vi "MDrive_PollingReadParam.vi"(4 "Device Name":string, 6 "Mdrive Mode":T2, 8 "error in (no error)":errorcluster, 10 "Get Parameter":T1, 11 "VISA Refnum in":refnum<visa-resource-name>) -> (0 "error out":errorcluster, 1 "String":string, 2 "Value":i32, 3 "VISA Refnum out":refnum<visa-resource-name>)   [LabVIEW 2015]
uses:
  MDrive Mode.ctl
  Get Parameter.ctl
  Stream/LP Globals.vi
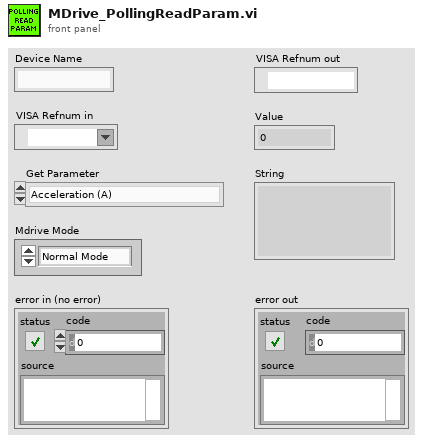
[diagram p1: front panel]
types:
  T1 = typedef "Get Parameter.ctl" = enum16{"Acceleration (A)", "Baud Rate (BD)", "Busy Flag (BY)", "Counter 1 (C1)", "Counter 2 (C2)", "Check Sum Enable (CK)", "Clock Mode (CM)", "Clock Mode Ratio (CR)", "Clock Mode Out Step Width (CW)", "Deceleration (D)", "Digital Filtering, Input 1 (D1)", "Digital Filtering, Input 2 (D2)", "Digital Filtering, Input 3 (D3)", "Digital Filtering, Input 4 (D4)", "Digital Filtering, Input 5 (D5)", "Digital Filtering, Input 9 (D9)", "Digital Filtering, Input 10 (D10)", "Digital Filtering, Input 11 (D11)", "Digital Filtering, Input 12 (D12)", "Deadband (DB)", "Enable/Disable Drive (DE)", "Device Name (DN)", "End Program Execution (E)", "Encoder Function Enable (EE)", "Encoder Lines (EL)", "Error Flag (EF)", "Error Variable (ER)", "Echo Mode (EM)", "Escape (ES)", "Execute Program at Address (EX)", "Hold Current (HC)", "Hold Current Delay Time (HI)", "Input 1 (I1)", "Input 2 (I2)", "Input 3 (I3)", "Input 4 (I4)", "Input 5 Analog (I5)", "Input 6 Encoder Index (I6)", "Input 9 (I9)", "Input 10 (I10)", "Input 11 (I11)", "Input 12 (I12)", "Input Low Byte (1-4) (IL)", "Input High Byte (9-12) (IH)", "Inputs Total (1-4,9-12) (IN)", "Internal Temperature (IT)", "Jog Enable (JE)", "Limit Stop Mode (LM)", "MicroStepping Select (MS)", "Motor Settling Delay Time (MT)", "Moving Flag (MV)", "Output 1 (O1)", "Output 2 (O2)", "Output 3 (O3)", "Output 4 (O4)", "Output 9 (O9)", "Output 10 (O10)", "Output 11 (O11)", "Output 12 (O12)", "Output High Byte (9-12) (OH)", "Output Low Byte (1-4) (OL)", "Output Total (1-4 and 9-12) (OT)", "Position (P)", "Position Captured at Trip (PC)", "Position Maintenance (PM)", "Part Number (PN)", "Party Mode (PY)", "Register 1 (R1)", "Register 2 (R2)", "Register 3 (R3)", "Register 4 (R4)", "Run Current (RC)", "Serial Number (SN)", "Stall Flag (ST)", "Stall Factor (SF)", "Stall Mode Set (SM)", "User Variables (UV)", "Velocity (V)", "Velocity Changing Flag (VC)", "Velocity Initial (VI)", "Version, Firmware (VR)", "Velocity Maximum (VM)", "Read Input1", "Read Input2"}
  T2 = typedef "MDrive Mode.ctl" = enum16{"Normal Mode", "Party Mode"}
  T3 = typedef "Semaphore RefNum" = refnum<k1>
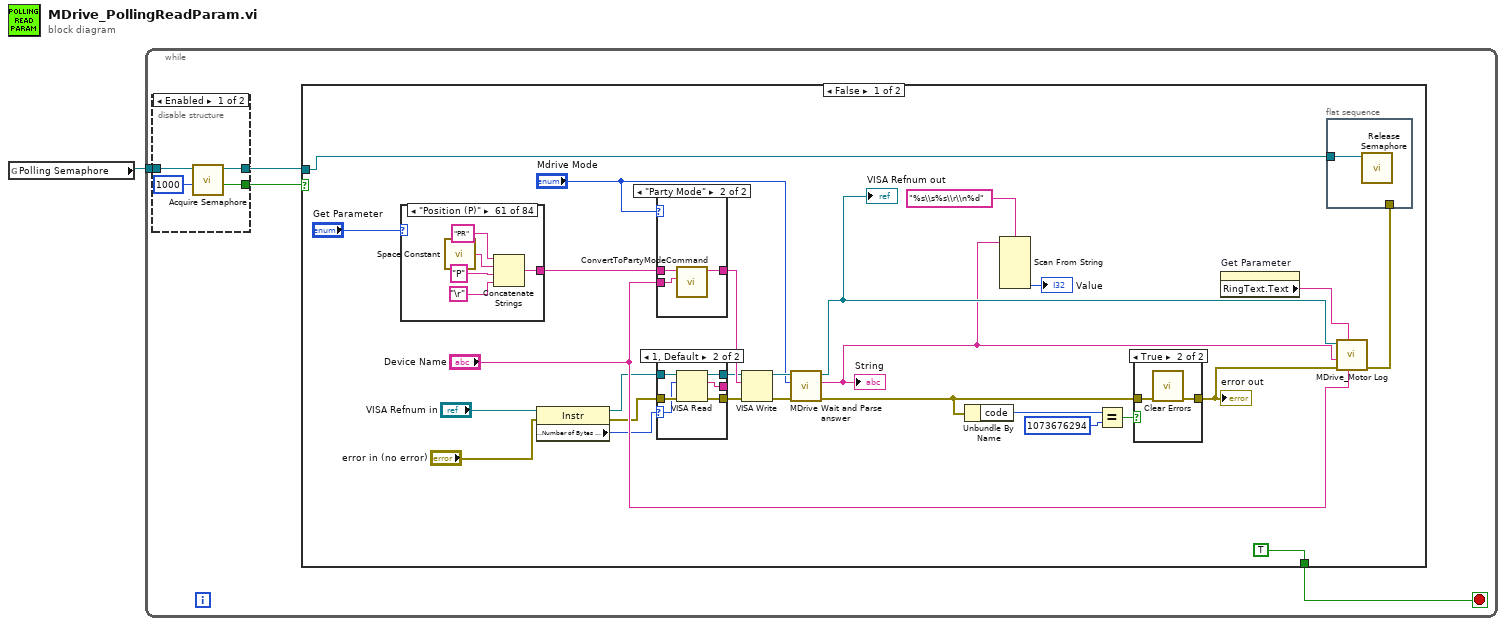
[diagram p0: block diagram]
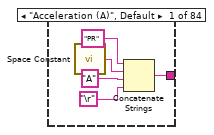
[diagram p5: hidden frame]
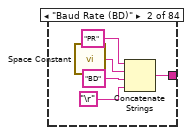
[diagram p6: hidden frame]
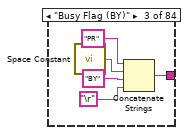
[diagram p7: hidden frame]
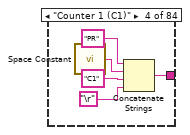
[diagram p8: hidden frame]
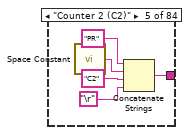
[diagram p9: hidden frame]
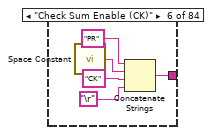
[diagram p10: hidden frame]
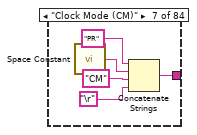
[diagram p11: hidden frame]
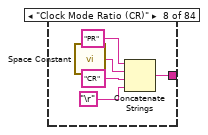
[diagram p12: hidden frame]
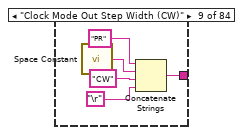
[diagram p13: hidden frame]
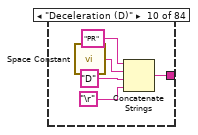
[diagram p14: hidden frame]
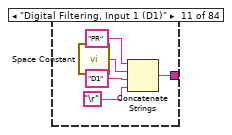
[diagram p15: hidden frame]
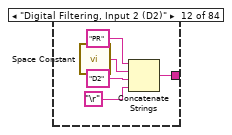
[diagram p16: hidden frame]
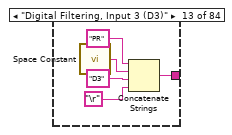
[diagram p17: hidden frame]
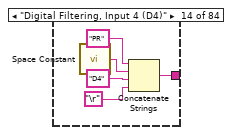
[diagram p18: hidden frame]
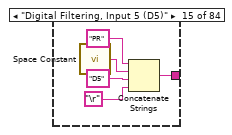
[diagram p19: hidden frame]
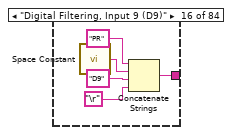
[diagram p20: hidden frame]
diagram:
  n1 = global read "LP Globals.vi" "Polling Semaphore"() -> (w1:T3)
  n2 = while {
    tunnel: w1 -> [w5]
    stop <- w4 stop-if-true
    n3 = disable-structure shown="Enabled" {
      disable-tunnel: w5 -> [w9 w10]
      disable-tunnel: [w7 w10] -> w3
      disable-tunnel: [w6 _] -> w2
      frame Enabled {
        n4 = call <vilib>:"Acquire Semaphore.vi"("ms timeout (-1)"=1000, "semaphore"=w9) -> ("timed out"=w6:bool, "semaphore out"=w7:T3)  [unwired: 3 in, 1 out]
      }
      frame Disabled {
      }
    }
    n5 = case shown="False" w2 {
      tunnel: [TRUE _] -> w4
      tunnel: w3 -> [w12 _]
      frame False {
        n6 = case shown="\"Position (P)\"" "Get Parameter" {
          tunnel: [w51 w56 w61 w66 w71 w76 w81 w86 w91 w96 w101 w106 w111 w116 w121 w126 w131 w136 w141 w146 w151 w156 w161 w166 w171 w176 w181 w186 w191 w196 w201 w206 w211 w216 w221 w226 w231 w236 w241 w246 w251 w256 w261 w266 w271 w276 w281 w286 w291 w296 w301 w306 w311 w316 w321 w326 w331 w336 w341 w346 w351 w356 w361 w366 w371 w376 w381 w386 w391 w396 w401 w406 w411 w416 w421 w426 w431 w436 w441 w446 w451 w456 w461 w466] -> w22
          frame "Acceleration (A)", Default {
            n7 = call <vilib>:"Space Constant.vi"() -> ("String"=w54:string)
            n8 = Concatenate Strings("PR" ("string"), w54, "A" ("string"), "\r") -> (w51:string)
          }
          frame "Baud Rate (BD)" {
            n9 = call <vilib>:"Space Constant.vi"() -> ("String"=w59:string)
            n10 = Concatenate Strings("PR" ("string"), w59, "BD" ("string"), "\r") -> (w56:string)
          }
          frame "Busy Flag (BY)" {
            n11 = call <vilib>:"Space Constant.vi"() -> ("String"=w64:string)
            n12 = Concatenate Strings("PR" ("string"), w64, "BY" ("string"), "\r") -> (w61:string)
          }
          frame "Counter 1 (C1)" {
            n13 = call <vilib>:"Space Constant.vi"() -> ("String"=w69:string)
            n14 = Concatenate Strings("PR" ("string"), w69, "C1" ("string"), "\r") -> (w66:string)
          }
          frame "Counter 2 (C2)" {
            n15 = call <vilib>:"Space Constant.vi"() -> ("String"=w74:string)
            n16 = Concatenate Strings("PR" ("string"), w74, "C2" ("string"), "\r") -> (w71:string)
          }
          frame "Check Sum Enable (CK)" {
            n17 = call <vilib>:"Space Constant.vi"() -> ("String"=w79:string)
            n18 = Concatenate Strings("PR" ("string"), w79, "CK" ("string"), "\r") -> (w76:string)
          }
          frame "Clock Mode (CM)" {
            n19 = call <vilib>:"Space Constant.vi"() -> ("String"=w84:string)
            n20 = Concatenate Strings("PR" ("string"), w84, "CM" ("string"), "\r") -> (w81:string)
          }
          frame "Clock Mode Ratio (CR)" {
            n21 = call <vilib>:"Space Constant.vi"() -> ("String"=w89:string)
            n22 = Concatenate Strings("PR" ("string"), w89, "CR" ("string"), "\r") -> (w86:string)
          }
          frame "Clock Mode Out Step Width (CW)" {
            n23 = call <vilib>:"Space Constant.vi"() -> ("String"=w94:string)
            n24 = Concatenate Strings("PR" ("string"), w94, "CW" ("string"), "\r") -> (w91:string)
          }
          frame "Deceleration (D)" {
            n25 = call <vilib>:"Space Constant.vi"() -> ("String"=w99:string)
            n26 = Concatenate Strings("PR" ("string"), w99, "D" ("string"), "\r") -> (w96:string)
          }
          frame "Digital Filtering, Input 1 (D1)" {
            n27 = call <vilib>:"Space Constant.vi"() -> ("String"=w104:string)
            n28 = Concatenate Strings("PR" ("string"), w104, "D1" ("string"), "\r") -> (w101:string)
          }
          frame "Digital Filtering, Input 2 (D2)" {
            n29 = call <vilib>:"Space Constant.vi"() -> ("String"=w109:string)
            n30 = Concatenate Strings("PR" ("string"), w109, "D2" ("string"), "\r") -> (w106:string)
          }
          frame "Digital Filtering, Input 3 (D3)" {
            n31 = call <vilib>:"Space Constant.vi"() -> ("String"=w114:string)
            n32 = Concatenate Strings("PR" ("string"), w114, "D3" ("string"), "\r") -> (w111:string)
          }
          frame "Digital Filtering, Input 4 (D4)" {
            n33 = call <vilib>:"Space Constant.vi"() -> ("String"=w119:string)
            n34 = Concatenate Strings("PR" ("string"), w119, "D4" ("string"), "\r") -> (w116:string)
          }
          frame "Digital Filtering, Input 5 (D5)" {
            n35 = call <vilib>:"Space Constant.vi"() -> ("String"=w124:string)
            n36 = Concatenate Strings("PR" ("string"), w124, "D5" ("string"), "\r") -> (w121:string)
          }
          frame "Digital Filtering, Input 9 (D9)" {
            n37 = call <vilib>:"Space Constant.vi"() -> ("String"=w129:string)
            n38 = Concatenate Strings("PR" ("string"), w129, "D9" ("string"), "\r") -> (w126:string)
          }
          frame "Digital Filtering, Input 10 (D10)" {
            n39 = call <vilib>:"Space Constant.vi"() -> ("String"=w134:string)
            n40 = Concatenate Strings("PR" ("string"), w134, "D10" ("string"), "\r") -> (w131:string)
          }
          frame "Digital Filtering, Input 11 (D11)" {
            n41 = call <vilib>:"Space Constant.vi"() -> ("String"=w139:string)
            n42 = Concatenate Strings("PR" ("string"), w139, "D11" ("string"), "\r") -> (w136:string)
          }
          frame "Digital Filtering, Input 12 (D12)" {
            n43 = call <vilib>:"Space Constant.vi"() -> ("String"=w144:string)
            n44 = Concatenate Strings("PR" ("string"), w144, "D12" ("string"), "\r") -> (w141:string)
          }
          frame "Deadband (DB)" {
            n45 = call <vilib>:"Space Constant.vi"() -> ("String"=w149:string)
            n46 = Concatenate Strings("PR" ("string"), w149, "DB" ("string"), "\r") -> (w146:string)
          }
          frame "Enable/Disable Drive (DE)" {
            n47 = call <vilib>:"Space Constant.vi"() -> ("String"=w154:string)
            n48 = Concatenate Strings("PR" ("string"), w154, "DE" ("string"), "\r") -> (w151:string)
          }
          frame "Device Name (DN)" {
            n49 = call <vilib>:"Space Constant.vi"() -> ("String"=w159:string)
            n50 = Concatenate Strings("PR" ("string"), w159, "DN" ("string"), "\r") -> (w156:string)
          }
          frame "End Program Execution (E)" {
            n51 = call <vilib>:"Space Constant.vi"() -> ("String"=w164:string)
            n52 = Concatenate Strings("PR" ("string"), w164, "E" ("string"), "\r") -> (w161:string)
          }
          frame "Encoder Function Enable (EE)" {
            n53 = call <vilib>:"Space Constant.vi"() -> ("String"=w169:string)
            n54 = Concatenate Strings("PR" ("string"), w169, "EE" ("string"), "\r") -> (w166:string)
          }
          frame "Error Flag (EF)" {
            n55 = call <vilib>:"Space Constant.vi"() -> ("String"=w174:string)
            n56 = Concatenate Strings("PR" ("string"), w174, "EF" ("string"), "\r") -> (w171:string)
          }
          frame "Error Variable (ER)" {
            n57 = call <vilib>:"Space Constant.vi"() -> ("String"=w179:string)
            n58 = Concatenate Strings("PR" ("string"), w179, "ER" ("string"), "\r") -> (w176:string)
          }
          frame "Echo Mode (EM)" {
            n59 = call <vilib>:"Space Constant.vi"() -> ("String"=w184:string)
            n60 = Concatenate Strings("PR" ("string"), w184, "EM" ("string"), "\r") -> (w181:string)
          }
          frame "Escape (ES)" {
            n61 = call <vilib>:"Space Constant.vi"() -> ("String"=w189:string)
            n62 = Concatenate Strings("PR" ("string"), w189, "ES" ("string"), "\r") -> (w186:string)
          }
          frame "Execute Program at Address (EX)" {
            n63 = call <vilib>:"Space Constant.vi"() -> ("String"=w194:string)
            n64 = Concatenate Strings("PR" ("string"), w194, "EX" ("string"), "\r") -> (w191:string)
          }
          frame "Hold Current (HC)" {
            n65 = call <vilib>:"Space Constant.vi"() -> ("String"=w199:string)
            n66 = Concatenate Strings("PR" ("string"), w199, "HC" ("string"), "\r") -> (w196:string)
          }
          frame "Hold Current Delay Time (HI)" {
            n67 = call <vilib>:"Space Constant.vi"() -> ("String"=w204:string)
            n68 = Concatenate Strings("PR" ("string"), w204, "HI" ("string"), "\r") -> (w201:string)
          }
          frame "Input 1 (I1)" {
            n69 = call <vilib>:"Space Constant.vi"() -> ("String"=w209:string)
            n70 = Concatenate Strings("PR" ("string"), w209, "I1" ("string"), "\r") -> (w206:string)
          }
          frame "Input 2 (I2)" {
            n71 = call <vilib>:"Space Constant.vi"() -> ("String"=w214:string)
            n72 = Concatenate Strings("PR" ("string"), w214, "I2" ("string"), "\r") -> (w211:string)
          }
          frame "Input 3 (I3)" {
            n73 = call <vilib>:"Space Constant.vi"() -> ("String"=w219:string)
            n74 = Concatenate Strings("PR" ("string"), w219, "I3" ("string"), "\r") -> (w216:string)
          }
          frame "Input 4 (I4)" {
            n75 = call <vilib>:"Space Constant.vi"() -> ("String"=w224:string)
            n76 = Concatenate Strings("PR" ("string"), w224, "I4" ("string"), "\r") -> (w221:string)
          }
          frame "Input 5 Analog (I5)" {
            n77 = call <vilib>:"Space Constant.vi"() -> ("String"=w229:string)
            n78 = Concatenate Strings("PR" ("string"), w229, "I5" ("string"), "\r") -> (w226:string)
          }
          frame "Input 6 Encoder Index (I6)" {
            n79 = call <vilib>:"Space Constant.vi"() -> ("String"=w234:string)
            n80 = Concatenate Strings("PR" ("string"), w234, "I6" ("string"), "\r") -> (w231:string)
          }
          frame "Input 9 (I9)" {
            n81 = call <vilib>:"Space Constant.vi"() -> ("String"=w239:string)
            n82 = Concatenate Strings("PR" ("string"), w239, "I9" ("string"), "\r") -> (w236:string)
          }
          frame "Input 10 (I10)" {
            n83 = call <vilib>:"Space Constant.vi"() -> ("String"=w244:string)
            n84 = Concatenate Strings("PR" ("string"), w244, "I10" ("string"), "\r") -> (w241:string)
          }
          frame "Input 11 (I11)" {
            n85 = call <vilib>:"Space Constant.vi"() -> ("String"=w249:string)
            n86 = Concatenate Strings("PR" ("string"), w249, "I3" ("string"), "\r") -> (w246:string)
          }
          frame "Input 12 (I12)" {
            n87 = call <vilib>:"Space Constant.vi"() -> ("String"=w254:string)
            n88 = Concatenate Strings("PR" ("string"), w254, "I12" ("string"), "\r") -> (w251:string)
          }
          frame "Input Low Byte (1-4) (IL)" {
            n89 = call <vilib>:"Space Constant.vi"() -> ("String"=w259:string)
            n90 = Concatenate Strings("PR" ("string"), w259, "IL" ("string"), "\r") -> (w256:string)
          }
          frame "Input High Byte (9-12) (IH)" {
            n91 = call <vilib>:"Space Constant.vi"() -> ("String"=w264:string)
            n92 = Concatenate Strings("PR" ("string"), w264, "IH" ("string"), "\r") -> (w261:string)
          }
          frame "Inputs Total (1-4,9-12) (IN)" {
            n93 = call <vilib>:"Space Constant.vi"() -> ("String"=w269:string)
            n94 = Concatenate Strings("PR" ("string"), w269, "IN" ("string"), "\r") -> (w266:string)
          }
          frame "Internal Temperature (IT)" {
            n95 = call <vilib>:"Space Constant.vi"() -> ("String"=w274:string)
            n96 = Concatenate Strings("PR" ("string"), w274, "IT" ("string"), "\r") -> (w271:string)
          }
          frame "Jog Enable (JE)" {
            n97 = call <vilib>:"Space Constant.vi"() -> ("String"=w279:string)
            n98 = Concatenate Strings("PR" ("string"), w279, "JE" ("string"), "\r") -> (w276:string)
          }
          frame "Limit Stop Mode (LM)" {
            n99 = call <vilib>:"Space Constant.vi"() -> ("String"=w284:string)
            n100 = Concatenate Strings("PR" ("string"), w284, "LM" ("string"), "\r") -> (w281:string)
          }
          frame "MicroStepping Select (MS)" {
            n101 = call <vilib>:"Space Constant.vi"() -> ("String"=w289:string)
            n102 = Concatenate Strings("PR" ("string"), w289, "MS" ("string"), "\r") -> (w286:string)
          }
          frame "Motor Settling Delay Time (MT)" {
            n103 = call <vilib>:"Space Constant.vi"() -> ("String"=w294:string)
            n104 = Concatenate Strings("PR" ("string"), w294, "MT" ("string"), "\r") -> (w291:string)
          }
          frame "Output 1 (O1)" {
            n105 = call <vilib>:"Space Constant.vi"() -> ("String"=w299:string)
            n106 = Concatenate Strings("PR" ("string"), w299, "O1" ("string"), "\r") -> (w296:string)
          }
          frame "Output 2 (O2)" {
            n107 = call <vilib>:"Space Constant.vi"() -> ("String"=w304:string)
            n108 = Concatenate Strings("PR" ("string"), w304, "O2" ("string"), "\r") -> (w301:string)
          }
          frame "Output 3 (O3)" {
            n109 = call <vilib>:"Space Constant.vi"() -> ("String"=w309:string)
            n110 = Concatenate Strings("PR" ("string"), w309, "O3" ("string"), "\r") -> (w306:string)
          }
          frame "Output 4 (O4)" {
            n111 = call <vilib>:"Space Constant.vi"() -> ("String"=w314:string)
            n112 = Concatenate Strings("PR" ("string"), w314, "O4" ("string"), "\r") -> (w311:string)
          }
          frame "Output 9 (O9)" {
            n113 = call <vilib>:"Space Constant.vi"() -> ("String"=w319:string)
            n114 = Concatenate Strings("PR" ("string"), w319, "O9" ("string"), "\r") -> (w316:string)
          }
          frame "Output 10 (O10)" {
            n115 = call <vilib>:"Space Constant.vi"() -> ("String"=w324:string)
            n116 = Concatenate Strings("PR" ("string"), w324, "O10" ("string"), "\r") -> (w321:string)
          }
          frame "Output 11 (O11)" {
            n117 = call <vilib>:"Space Constant.vi"() -> ("String"=w329:string)
            n118 = Concatenate Strings("PR" ("string"), w329, "O11" ("string"), "\r") -> (w326:string)
          }
          frame "Output 12 (O12)" {
            n119 = call <vilib>:"Space Constant.vi"() -> ("String"=w334:string)
            n120 = Concatenate Strings("PR" ("string"), w334, "O12" ("string"), "\r") -> (w331:string)
          }
          frame "Output High Byte (9-12) (OH)" {
            n121 = call <vilib>:"Space Constant.vi"() -> ("String"=w339:string)
            n122 = Concatenate Strings("PR" ("string"), w339, "OH" ("string"), "\r") -> (w336:string)
          }
          frame "Output Low Byte (1-4) (OL)" {
            n123 = call <vilib>:"Space Constant.vi"() -> ("String"=w344:string)
            n124 = Concatenate Strings("PR" ("string"), w344, "OL" ("string"), "\r") -> (w341:string)
          }
          frame "Output Total (1-4 and 9-12) (OT)" {
            n125 = call <vilib>:"Space Constant.vi"() -> ("String"=w349:string)
            n126 = Concatenate Strings("PR" ("string"), w349, "OT" ("string"), "\r") -> (w346:string)
          }
          frame "Position (P)" {
            n127 = call <vilib>:"Space Constant.vi"() -> ("String"=w354:string)
            n128 = Concatenate Strings("PR" ("string"), w354, "P" ("string"), "\r") -> (w351:string)
          }
          frame "Position Captured at Trip (PC)" {
            n129 = call <vilib>:"Space Constant.vi"() -> ("String"=w359:string)
            n130 = Concatenate Strings("PR" ("string"), w359, "PC" ("string"), "\r") -> (w356:string)
          }
          frame "Position Maintenance (PM)" {
            n131 = call <vilib>:"Space Constant.vi"() -> ("String"=w364:string)
            n132 = Concatenate Strings("PR" ("string"), w364, "PM" ("string"), "\r") -> (w361:string)
          }
          frame "Part Number (PN)" {
            n133 = call <vilib>:"Space Constant.vi"() -> ("String"=w369:string)
            n134 = Concatenate Strings("PR" ("string"), w369, "PN" ("string"), "\r") -> (w366:string)
          }
          frame "Party Mode (PY)" {
            n135 = call <vilib>:"Space Constant.vi"() -> ("String"=w374:string)
            n136 = Concatenate Strings("PR" ("string"), w374, "PY" ("string"), "\r") -> (w371:string)
          }
          frame "Register 1 (R1)" {
            n137 = call <vilib>:"Space Constant.vi"() -> ("String"=w379:string)
            n138 = Concatenate Strings("PR" ("string"), w379, "R1" ("string"), "\r") -> (w376:string)
          }
          frame "Register 2 (R2)" {
            n139 = call <vilib>:"Space Constant.vi"() -> ("String"=w384:string)
            n140 = Concatenate Strings("PR" ("string"), w384, "R2" ("string"), "\r") -> (w381:string)
          }
          frame "Register 3 (R3)" {
            n141 = call <vilib>:"Space Constant.vi"() -> ("String"=w389:string)
            n142 = Concatenate Strings("PR" ("string"), w389, "R3" ("string"), "\r") -> (w386:string)
          }
          frame "Register 4 (R4)" {
            n143 = call <vilib>:"Space Constant.vi"() -> ("String"=w394:string)
            n144 = Concatenate Strings("PR" ("string"), w394, "R4" ("string"), "\r") -> (w391:string)
          }
          frame "Run Current (RC)" {
            n145 = call <vilib>:"Space Constant.vi"() -> ("String"=w399:string)
            n146 = Concatenate Strings("PR" ("string"), w399, "RC" ("string"), "\r") -> (w396:string)
          }
          frame "Serial Number (SN)" {
            n147 = call <vilib>:"Space Constant.vi"() -> ("String"=w404:string)
            n148 = Concatenate Strings("PR" ("string"), w404, "SN" ("string"), "\r") -> (w401:string)
          }
          frame "Stall Flag (ST)" {
            n149 = call <vilib>:"Space Constant.vi"() -> ("String"=w409:string)
            n150 = Concatenate Strings("PR" ("string"), w409, "ST" ("string"), "\r") -> (w406:string)
          }
          frame "Stall Factor (SF)" {
            n151 = call <vilib>:"Space Constant.vi"() -> ("String"=w414:string)
            n152 = Concatenate Strings("PR" ("string"), w414, "SF" ("string"), "\r") -> (w411:string)
          }
          frame "Stall Mode Set (SM)" {
            n153 = call <vilib>:"Space Constant.vi"() -> ("String"=w419:string)
            n154 = Concatenate Strings("PR" ("string"), w419, "SM" ("string"), "\r") -> (w416:string)
          }
          frame "User Variables (UV)" {
            n155 = call <vilib>:"Space Constant.vi"() -> ("String"=w424:string)
            n156 = Concatenate Strings("PR" ("string"), w424, "UV" ("string"), "\r") -> (w421:string)
          }
          frame "Velocity (V)" {
            n157 = call <vilib>:"Space Constant.vi"() -> ("String"=w429:string)
            n158 = Concatenate Strings("PR" ("string"), w429, "V" ("string"), "\r") -> (w426:string)
          }
          frame "Velocity Changing Flag (VC)" {
            n159 = call <vilib>:"Space Constant.vi"() -> ("String"=w434:string)
            n160 = Concatenate Strings("PR" ("string"), w434, "VC" ("string"), "\r") -> (w431:string)
          }
          frame "Velocity Initial (VI)" {
            n161 = call <vilib>:"Space Constant.vi"() -> ("String"=w439:string)
            n162 = Concatenate Strings("PR" ("string"), w439, "VI" ("string"), "\r") -> (w436:string)
          }
          frame "Version, Firmware (VR)" {
            n163 = call <vilib>:"Space Constant.vi"() -> ("String"=w444:string)
            n164 = Concatenate Strings("PR" ("string"), w444, "VR" ("string"), "\r") -> (w441:string)
          }
          frame "Velocity Maximum (VM)" {
            n165 = call <vilib>:"Space Constant.vi"() -> ("String"=w449:string)
            n166 = Concatenate Strings("PR" ("string"), w449, "VM" ("string"), "\r") -> (w446:string)
          }
          frame "Moving Flag (MV)" {
            n167 = call <vilib>:"Space Constant.vi"() -> ("String"=w454:string)
            n168 = Concatenate Strings("PR" ("string"), w454, "MV" ("string"), "\r") -> (w451:string)
          }
          frame "Encoder Lines (EL)" {
            n169 = call <vilib>:"Space Constant.vi"() -> ("String"=w459:string)
            n170 = Concatenate Strings("PR" ("string"), w459, "EL" ("string"), "\r") -> (w456:string)
          }
          frame "Read Input1" {
            n171 = call <vilib>:"Space Constant.vi"() -> ("String"=w464:string)
            n172 = Concatenate Strings("PR" ("string"), w464, "I1" ("string"), "\r") -> (w461:string)
          }
          frame "Read Input2" {
            n173 = call <vilib>:"Space Constant.vi"() -> ("String"=w469:string)
            n174 = Concatenate Strings("PR" ("string"), w469, "I2" ("string"), "\r") -> (w466:string)
          }
        }
        n175 = property class="Instr"(reference="VISA Refnum in", error in="error in (no error)") -> (reference out=w18:refnum<visa-resource-name>, error out=w17:errorcluster, "Serial Settings:Number of Bytes at Serial Port"=w16:u32)
        n176 = case shown="\"Party Mode\"" "Mdrive Mode" {
          tunnel: "Device Name" -> [_ w50]
          tunnel: w22 -> [w47 w49]
          tunnel: [w47 w48] -> w28
          frame "Normal Mode", Default {
          }
          frame "Party Mode" {
            n177 = call "ConvertToPartyModeCommand.vi"("Device Name"=w50, "Command"=w49) -> ("Command out"=w48:string)  [unwired: 9 in]
          }
        }
        n178 = case shown="1, Default" w16 {
          selector: w16 -> [_ w42]
          tunnel: [w40 w46] -> w27
          tunnel: [w39 w45] -> w26
          tunnel: w18 -> [w40 w44]
          tunnel: w17 -> [w39 w43]
          tunnel: [_ w41] -> _
          frame 0 {
          }
          frame 1, Default {
            n179 = VISA Read(VISA resource name=w44, byte count=w42, error in (no error)=w43) -> (VISA resource name out=w46:refnum<visa-resource-name>, read buffer=w41:string, error out=w45:errorcluster)  [unwired: 1 out]
          }
        }
        n180 = VISA Write(VISA resource name=w27, write buffer=w28, error in (no error)=w26) -> (VISA resource name out=w30:refnum<visa-resource-name>, error out=w29:errorcluster)  [unwired: 1 out]
        n181 = call "MDrive Wait and Parse answer.vi"("error in (no error)"=w29, "Mdrive Mode"="Mdrive Mode", "VISA Refnum in"=w30) -> ("error out"=w37:errorcluster, "String"=w15:string, "VISA Refnum out"=w33:refnum<visa-resource-name>)  [unwired: 6 in]
        "String" <- w15
        "VISA Refnum out" <- w33
        n182 = Unbundle By Name(w37) -> ("code"=w34:i32)
        n183 = Scan From String(format string="%s\\s%s\\r\\n%d", input string=w15) -> (output 3=→"Value":i32)  [unwired: 7 in, 3 out]
        n184 = Equal?(x=w34, y=1073676294 ("code")) -> (x = y?=w36:bool)
        n185 = case shown="True" w36 {
          tunnel: w37 -> [w471 w473]
          tunnel: [w471 w472] -> w24
          frame False {
          }
          frame True {
            n186 = call <vilib>:"Clear Errors.vi"("error in (no error)"=w473) -> ("error out"=w472:errorcluster)  [unwired: 5 in, 1 out]
          }
        }
        "error out" <- w24
        n187 = property on="Get Parameter" class="Enum (strict)"() -> ("RingText.Text"=w32:string)  [unwired: 2 in, 2 out]
        n188 = flat-sequence {
          tunnel: w12 -> [w38]
          tunnel: w11 -> [_]
          frame #0 {
            n189 = call <vilib>:"Release Semaphore.vi"("semaphore"=w38) -> ()  [unwired: 5 in, 2 out]
          }
        }
        n190 = call "MDrive_Motor Log.vi"("Motor Name"="Device Name", "Function"=w32, "Error in"=w24, "read buffer"=w15, "COM"=w33) -> ("Error out"=w11:errorcluster)  [unwired: 6 in]
      }
      frame True {
      }
    }
  }
